vi "User Interface.vi"(8 "error in (no error)":errorcluster, 11 "User Interface in":refnum<class "User Interface.lvclass">) -> (0 "error out":errorcluster, 3 "User Interface out":refnum<class "User Interface.lvclass">)   [LabVIEW 2017, in "DSF Core.lvlib" / "UDP Transfer Tx User Interface.lvclass"]
uses:
  UDP Transfer Tx User Interface.lvclass
  Classes/User Interface/User Interface.lvclass
  Configuration/Tx Transfer/UDP Transfer Tx Configuration.lvclass
  C:/Git/DSF/Core/Classes/Configuration/Configuration.lvclass
  Classes/Configuration/Configuration.lvclass
panel:
  in  "Destination Address":string
  in  "Destination Port":u16
  out "Data Version":string
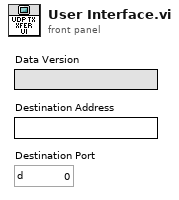
[diagram p1: front panel]
types:
  T1 = typedef "DSF Core.lvlib/UDP Transfer Tx Configuration.lvclass/Tx Transfer Settings.ctl" = cluster{"address":u32, "port":u16}
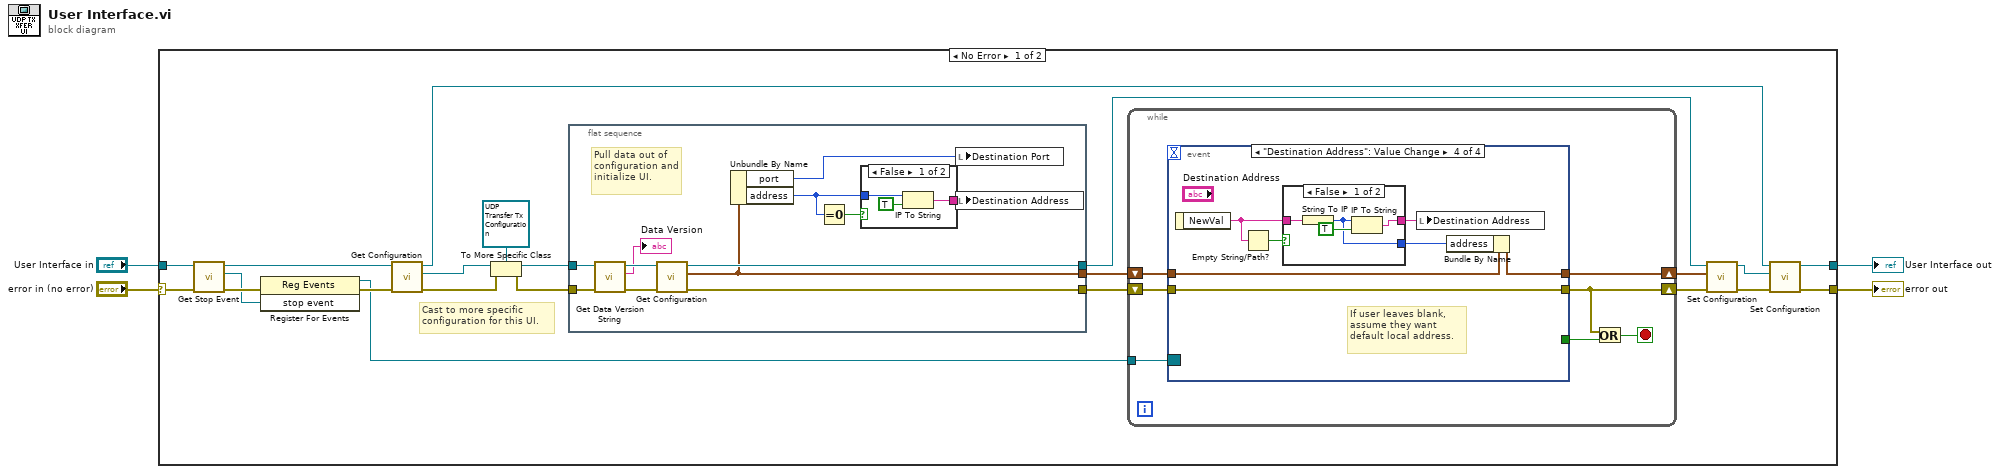
[diagram p0: block diagram]
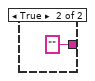
[diagram p2: hidden frame]
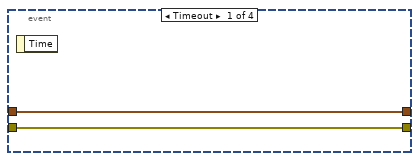
[diagram p3: hidden frame]
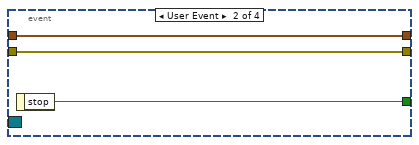
[diagram p4: hidden frame]
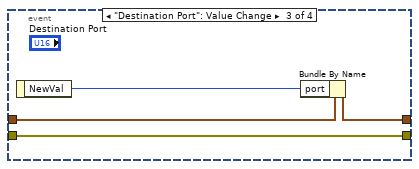
[diagram p5: hidden frame]
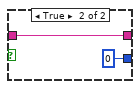
[diagram p6: hidden frame]
diagram:
  n1 = case shown="No Error" "error in (no error)" {
    selector: "error in (no error)" -> [w23 w73]
    tunnel: [w14 w73] -> w4
    tunnel: "User Interface in" -> [w22 w72]
    tunnel: [w13 w72] -> w1
    frame No Error {
      # "Cast to more specific configuration for this UI."
      n2 = call "Get Stop Event.vi"("error in (no error)"=w23, "User Interface in"=w22) -> ("error out"=w21:errorcluster, "stop event"=w20:refnum<user-event>, "User Interface out"=w19:refnum<class "User Interface.lvclass">)  [unwired: 7 in]
      n3 = register-events(error in=w21, w20) -> (reference out=w17:refnum<event-registration>, error out=w18:errorcluster)  [unwired: 1 in]
      n4 = call "Get Configuration.vi"("error in (no error)"=w18, "User Interface in"=w19) -> ("error out"=w16:errorcluster, "configuration"=w15:refnum<class "Configuration.lvclass">, "User Interface out"=w12:refnum<class "User Interface.lvclass">)  [unwired: 7 in]
      n5 = To More Specific Class(target class=refnum<class "UDP Transfer Tx Configuration.lvclass"> refnum ("DSF Core.lvlib:UDP Transfer Tx Configuration.lvclass"), reference=w15, error in=w16) -> (specific class reference=w26:refnum<class "UDP Transfer Tx Configuration.lvclass">, error out=w24:errorcluster)
      n6 = flat-sequence {
        tunnel: [w33] -> w25
        tunnel: w24 -> [w38]
        tunnel: w26 -> [w37]
        tunnel: [w30] -> w6
        tunnel: [w29] -> w10
        frame #0 {
          # "Pull data out of configuration and initialize UI."
          n7 = call "Get Data Version String.vi"("error in (no error)"=w38, "Configuration in"=w37) -> ("error out"=w36:errorcluster, "data version"=→"Data Version":string, "Configuration out"=w35:refnum<class "UDP Transfer Tx Configuration.lvclass">)  [unwired: 7 in]
          n8 = call "Get Configuration.vi"("error in (no error)"=w36, "UDP Transfer Tx Configuration in"=w35) -> ("error out"=w33:errorcluster, "transfer settings"=w29:T1, "UDP Transfer Tx Configuration out"=w30:refnum<class "UDP Transfer Tx Configuration.lvclass">)  [unwired: 7 in]
          n9 = Unbundle By Name(w29) -> ("port"=w32:u16, "address"=w28:u32)
          n10 = Equal To 0?(x=w28) -> (x = 0?=w27:bool)
          n11 = case shown="False" w27 {
            tunnel: [w41 "" ("name")] -> w31
            tunnel: w28 -> [w40 _]
            frame False {
              n12 = IP To String(1:TRUE ("dot notation? (F)"), 2:w40) -> (0:w41:string)
            }
            frame True {
            }
          }
          n13 = local write "Destination Port"(w32) -> ()
          n14 = local write "Destination Address"(w31) -> ()
        }
      }
      n15 = while {
        tunnel: w17 -> [w49]
        shift-right: [w47] -> w9
        shift-left: w25 -> [w48]
        shift-right: [w43] -> w7
        shift-left: w10 -> [w44]
        stop <- w46 stop-if-true
        n16 = event shown="[3] \"Destination Address\": Value Change" {
          selector: w49 -> [_ _ _ _]
          dyn-events: _ -> [_ _ _ _]
          timeout: _ -> [_ _ _ _]
          tunnel: [_ w53 _ _] -> w45
          tunnel: w48 -> [w51 w54 w58 w62]
          tunnel: [w51 w54 w58 w62] -> w47
          tunnel: w44 -> [w50 w52 w57 w63]
          tunnel: [w50 w52 w56 w65] -> w43
          event Timeout {
            n17 = event-data() -> ()  [unwired: 1 in, 1 out]
          }
          event User Event {
            n18 = event-data() -> ("stop"=w53:bool)  [unwired: 1 in]
          }
          event "Destination Port": Value Change {
            n19 = event-data() -> ("NewVal"=w55:u16)  [unwired: 1 in]
            n20 = Bundle By Name(cluster=w57, "port"=w55) -> (w56:T1)
          }
          event "Destination Address": Value Change {
            # "If user leaves blank, assume they want default local address."
            n21 = event-data() -> ("NewVal"=w60:string)  [unwired: 1 in]
            n22 = Empty String/Path?(string/path=w60) -> (empty?=w61:bool)
            n23 = case shown="False" w61 {
              tunnel: [w69 w70] -> w64
              tunnel: w60 -> [w68 w70]
              tunnel: [w66 u32 0] -> w59
              frame False {
                n24 = String To IP(1:w68) -> (0:w66:u32)
                n25 = IP To String(1:TRUE ("dot notation? (F)"), 2:w66) -> (0:w69:string)
              }
              frame True {
              }
            }
            n26 = local write "Destination Address"(w64) -> ()
            n27 = Bundle By Name(cluster=w63, "address"=w59) -> (w65:T1)
          }
        }
        n28 = Or(x=w47, y=w45) -> (x .or. y?=w46:bool)
      }
      n29 = call "Set Configuration.vi"("error in (no error)"=w9, "transfer settings"=w7, "UDP Transfer Tx Configuration in"=w6) -> ("error out"=w8:errorcluster, "UDP Transfer Tx Configuration out"=w5:refnum<class "UDP Transfer Tx Configuration.lvclass">)  [unwired: 7 in]
      n30 = call "Set Configuration.vi"("error in (no error)"=w8, "configuration"=w5, "User Interface in"=w12) -> ("error out"=w14:errorcluster, "User Interface out"=w13:refnum<class "User Interface.lvclass">)  [unwired: 7 in]
    }
    frame Error {
    }
  }
  "error out" <- w4
  "User Interface out" <- w1
